vi "demo.vi"() -> ()   [LabVIEW 2013]
uses:
  <vilib>/addons/_AddQ/G#Object/G#Object.lvclass
  Colleague_class/Colleague.lvclass
panel:
  in  "Device C to Device A":string
  in  "Device B to Device C":string
  out "Output":string
  in  "停止":bool
  in  "Device A to Device B":string
  out "# of objects killed":i32
  # "Device A"
  # "Device B"
  # "Device C"
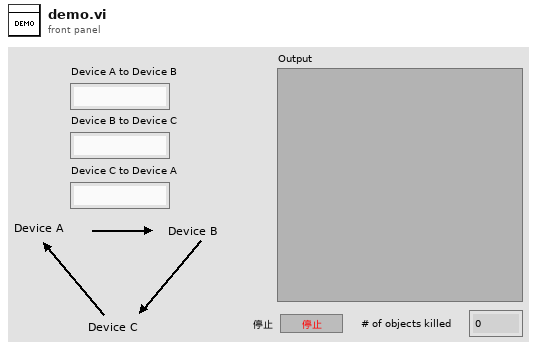
[diagram p1: front panel]
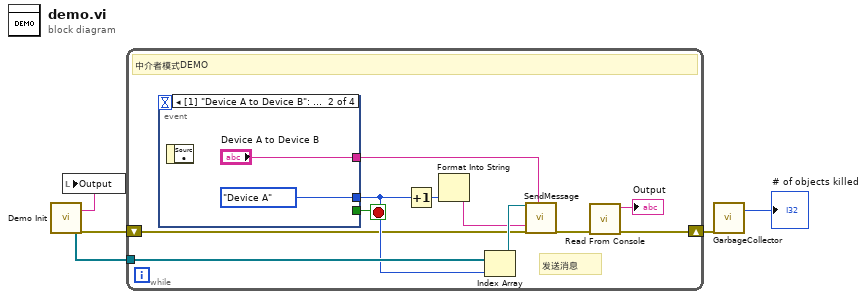
[diagram p0: block diagram]
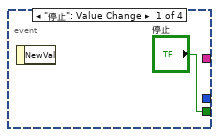
[diagram p2: hidden frame]
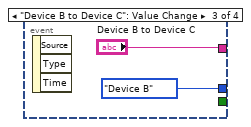
[diagram p3: hidden frame]
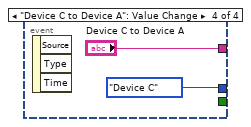
[diagram p4: hidden frame]
diagram:
  n1 = call "Demo Init.vi"() -> ("Colleague Array"=w3:refnum<class "Device.lvclass">[], "Output"=w2:string, "错误输出"=w1:errorcluster)  [unwired: 17 in]
  n2 = local write "Output"(w2) -> ()
  n3 = while {
    shift-right: [w7] -> w4
    shift-left: w1 -> [w9]
    tunnel: w3 -> [w15]
    stop <- w16 stop-if-true
    # "发送消息"
    # "中介者模式DEMO"
    n4 = event shown="[1] \"Device A to Device B\": 值改变" {
      selector: _ -> [_ _ _ _]
      dyn-events: _ -> [_ _ _ _]
      timeout: _ -> [_ _ _ _]
      tunnel: ["停止" _ _ _] -> w16
      tunnel: [_ enum16{"Device A", "Device B", "Device C"}."Device A" enum16{"Device A", "Device B", "Device C"}."Device B" enum16{"Device A", "Device B", "Device C"}."Device C"] -> w12
      tunnel: [_ "Device A to Device B" "Device B to Device C" "Device C to Device A"] -> w13
      event "停止": Value Change {
        n5 = event-data() -> ()  [unwired: 1 in, 1 out]
      }
      event "Device A to Device B": Value Change {
        n6 = event-data() -> ()  [unwired: 1 in, 1 out]
      }
      event "Device B to Device C": Value Change {
        n7 = event-data() -> ()  [unwired: 1 in, 3 out]
      }
      event "Device C to Device A": Value Change {
        n8 = event-data() -> ()  [unwired: 1 in, 3 out]
      }
    }
    n9 = Increment(x=w12) -> (x+1=w11:enum16{"Device A", "Device B", "Device C"})
    n10 = Format Into String(w11) -> (resulting string=w10:string)  [unwired: 3 in, 1 out]
    n11 = Index Array(array=w15, index=w12) -> (element=w14:refnum<class "Device.lvclass">)
    n12 = call "SendMessage.vi"("reference in"=w14, "Receiver"=w10, "error in (no error)"=w9, "Message"=w13) -> ("error out"=w8:errorcluster)  [unwired: 14 in, 1 out]
    n13 = call "Read From Console.vi"("error in (no error)"=w8) -> ("error out"=w7:errorcluster, "Output"=→"Output":string)  [unwired: 9 in]
  }
  n14 = call <vilib>:"GarbageCollector.vi"("error in (no error)"=w4) -> ("# of objects killed"=→"# of objects killed":i32)  [unwired: 16 in, 2 out]
